vi "HRTF-Configure Hardware (NI).vi"(0 "Params":T2={"Fs (Hz)"=0.0, "atten (dB)"=0.0, "Waveform"=enum."Chirp", "Freq Res (Hz)"=0.0, "Order"=0, "Averages"=0, "seed"=-1, "Window"={"Type"=enum."None", "Length (ms)"=0.0, "Center (ms)"=0.0}}, 7 "State":T1, 11 "error in (no error)":errorcluster) -> (4 "Stimulus":dbl[](array[numeric]), 6 "Sample Rate (Hz)":dbl, 8 "pts/rep":i32, 10 "reps/frame":i32, 15 "error out":errorcluster)   [LabVIEW 2015]
uses:
  Typedefs/HRTF-Parameters.ctl
  Typedefs/HRTF-Waveform.ctl
  Typedefs/HRTF-Window.ctl
  Typedefs/HRTF-Window Type.ctl
  Typedefs/HRTF-State.ctl
  Utility VIs/Math VIs/dB to Linear (scalar).vi
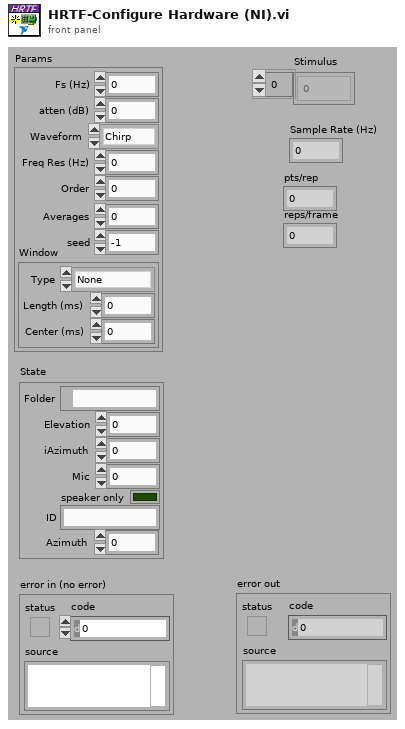
[diagram p1: front panel]
types:
  T1 = typedef "HRTF-State.ctl" = cluster{"Folder":path, "Elevation":dbl, "iAzimuth":i32, "Mic":i32, "speaker only":bool, "ID":string, "Azimuth":dbl}
  T2 = typedef "HRTF-Parameters.ctl" = cluster{"Fs (Hz)":dbl, "atten (dB)":dbl, "Waveform":T3, "Freq Res (Hz)":dbl, "Order":i32, "Averages":i32, "seed":i64, "Window":T4}
  T3 = typedef "HRTF-Waveform.ctl" = enum16{"Chirp", "MLS"}
  T4 = typedef "HRTF-Window.ctl" = cluster{"Type":T5, "Length (ms)":dbl, "Center (ms)":dbl}
  T5 = typedef "HRTF-Window Type.ctl" = enum16{"None", "Rectangle", "Hanning"}
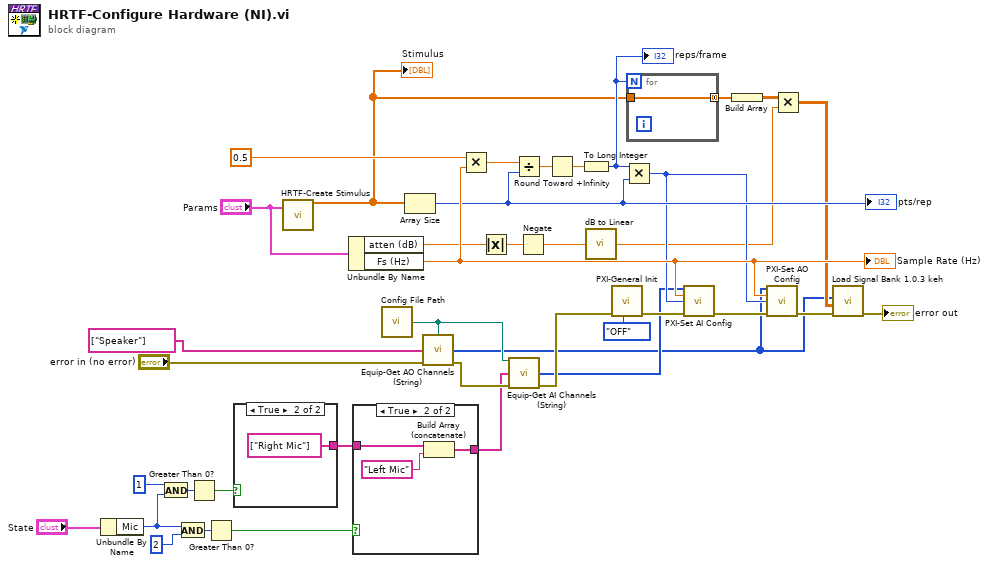
[diagram p0: block diagram]
diagram:
  n1 = Unbundle By Name("State") -> ("Mic"=w7:i32)
  n2 = And(x=1, y=w7) -> (x .and. y?=w9:i32)
  n3 = And(x=w7, y=2) -> (x .and. y?=w8:i32)
  n4 = Greater Than 0?(x=w9) -> (x > 0?=w4:bool)
  n5 = Greater Than 0?(x=w8) -> (x > 0?=w3:bool)
  n6 = case shown="True" w4 {
    tunnel: [_ string[] ["Right Mic"] ("Requested Endpoints")] -> w2
    frame False {
    }
    frame True {
    }
  }
  n7 = call "HRTF-Create Stimulus.vi"("Params"="Params") -> ("Stimulus"=w18:dbl[])  [unwired: 9 in, 5 out]
  "Stimulus" <- w18
  n8 = Unbundle By Name("Params") -> ("atten (dB)"=w22:dbl, "Fs (Hz)"=w31:dbl)
  "Sample Rate (Hz)" <- w31
  n9 = case shown="True" w3 {
    tunnel: w2 -> [w41 w44]
    tunnel: [w41 w42] -> w1
    frame False {
    }
    frame True {
      n10 = Build Array (concatenate)(w44, "Left Mic" ("String")) -> (w42:string[])
    }
  }
  n11 = call "Config File Path.vi"() -> ("Default config file name"=w15:path)  [unwired: 1 in]
  n12 = Array Size(array=w18) -> (size(s)=w29:i32)
  "pts/rep" <- w29
  n13 = call "Equip-Get AO Channels (String).vi"("Path"=w15, "Channel Names"=string[] ["Speaker"] ("Requested Endpoints"), "error in (no error)"="error in (no error)") -> ("AO Channels"=w11:i32[], "error out"=w14:errorcluster)  [unwired: 11 in]
  n14 = Multiply(x=0.5, y=w31) -> (x*y=w30:dbl)
  n15 = Absolute Value(x=w22) -> (abs(x)=w21:dbl)
  n16 = call "Equip-Get AI Channels (String).vi"("Path"=w15, "Inputs"=w1, "error in (no error)"=w14) -> ("AI Channels"=w12:i32[], "error out"=w13:errorcluster)  [unwired: 11 in]
  n17 = Divide(x=w30, y=w29) -> (x/y=w33:dbl)
  n18 = Negate(x=w21) -> (-x=w20:dbl)
  n19 = Round Toward +Infinity(x=w33) -> (ceil(x): smallest int >= x=w32:dbl)
  n20 = To Long Integer(number=w32) -> (32bit integer=w26:i32)
  "reps/frame" <- w26
  n21 = call-poly "dB to Linear.vi"("dB"=w20) -> ("linear"=w19:dbl)
  n22 = call "PXI-General Init.vi"("Double Buffer Mode"=enum32{"OFF", "ENABLED", "FORCED"}."OFF", "error in (no error)"=w13) -> ("error out"=w38:errorcluster)  [unwired: 9 in]
  n23 = Multiply(x=w26, y=w29) -> (x*y=w28:i32)
  n24 = for {
    N: w26 -> [_]
    tunnel: w18 -> [w45]
    tunnel: [w45] -> w25 mode=concatenating
  }
  n25 = call "PXI-Set AI Config.vi"("AI Channels"=w12, "Sampling Rate (Hz)"=w31, "Buffer Size"=w28, "error in (no error)"=w38) -> ("error out"=w37:errorcluster)  [unwired: 11 in]
  n26 = Build Array(w25) -> (w35:dbl[][])
  n27 = call "PXI-Set AO Config.vi"("AO Channels"=w11, "Sampling Rate (Hz)"=w31, "Buffer Size"=w28, "error in (no error)"=w37) -> ("error out"=w36:errorcluster)  [unwired: 11 in]
  n28 = Multiply(x=w35, y=w19) -> (x*y=w23:dbl[][])
  n29 = call "Load Signal Bank 1.0.3 keh.vi"("error in (no error)"=w36, "Input array"=w23, "Active AO Array"=w11) -> ("error out"=→"error out":errorcluster)  [unwired: 6 in, 2 out]
